vi "AB_860_900_Project_EXE_Info.vi"(7 "action":T1, 8 "error in (no error)":errorcluster, 10 "Exe_info in":T2, 11 "Object In":T3) -> (0 "error out":errorcluster, 2 "Exe info out":T2, 3 "Object Out":T3)   [LabVIEW 2020]
uses:
  <resource>/Framework/Providers/API/ItemRef.ctl
  <vilib>/AppBuilder/RW_Project/AB_RW_Project_PropBag_Action.ctl
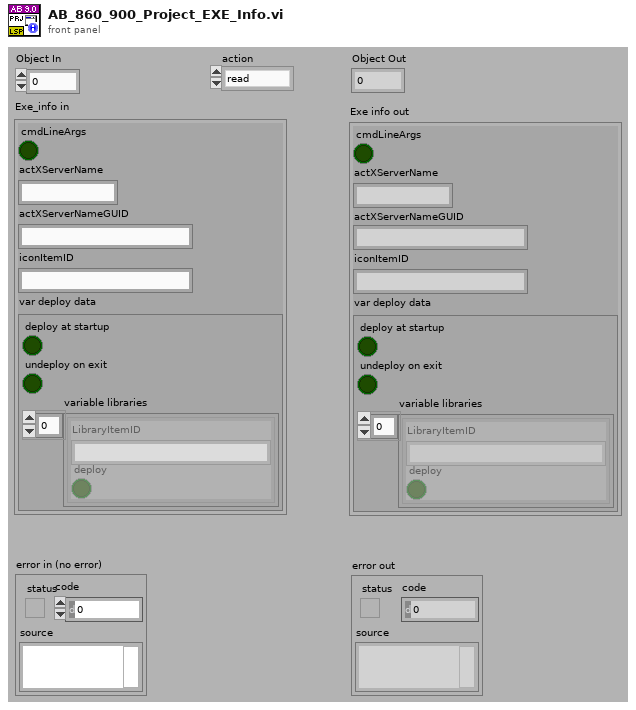
[diagram p1: front panel]
types:
  T1 = typedef "AB_RW_Project_PropBag_Action.ctl" = enum16{"read", "write", "clear", "readPrevious", "writePrevious", "clearPrevious"}
  T2 = cluster{"cmdLineArgs":bool, "actXServerName":string, "actXServerNameGUID":string, "iconItemID":string, "var deploy data":cluster{"deploy at startup":bool, "undeploy on exit":bool, "variable libraries":cluster{"LibraryItemID":string, "deploy":bool}[]}}
  T3 = typedef "ItemRef.ctl" = u64
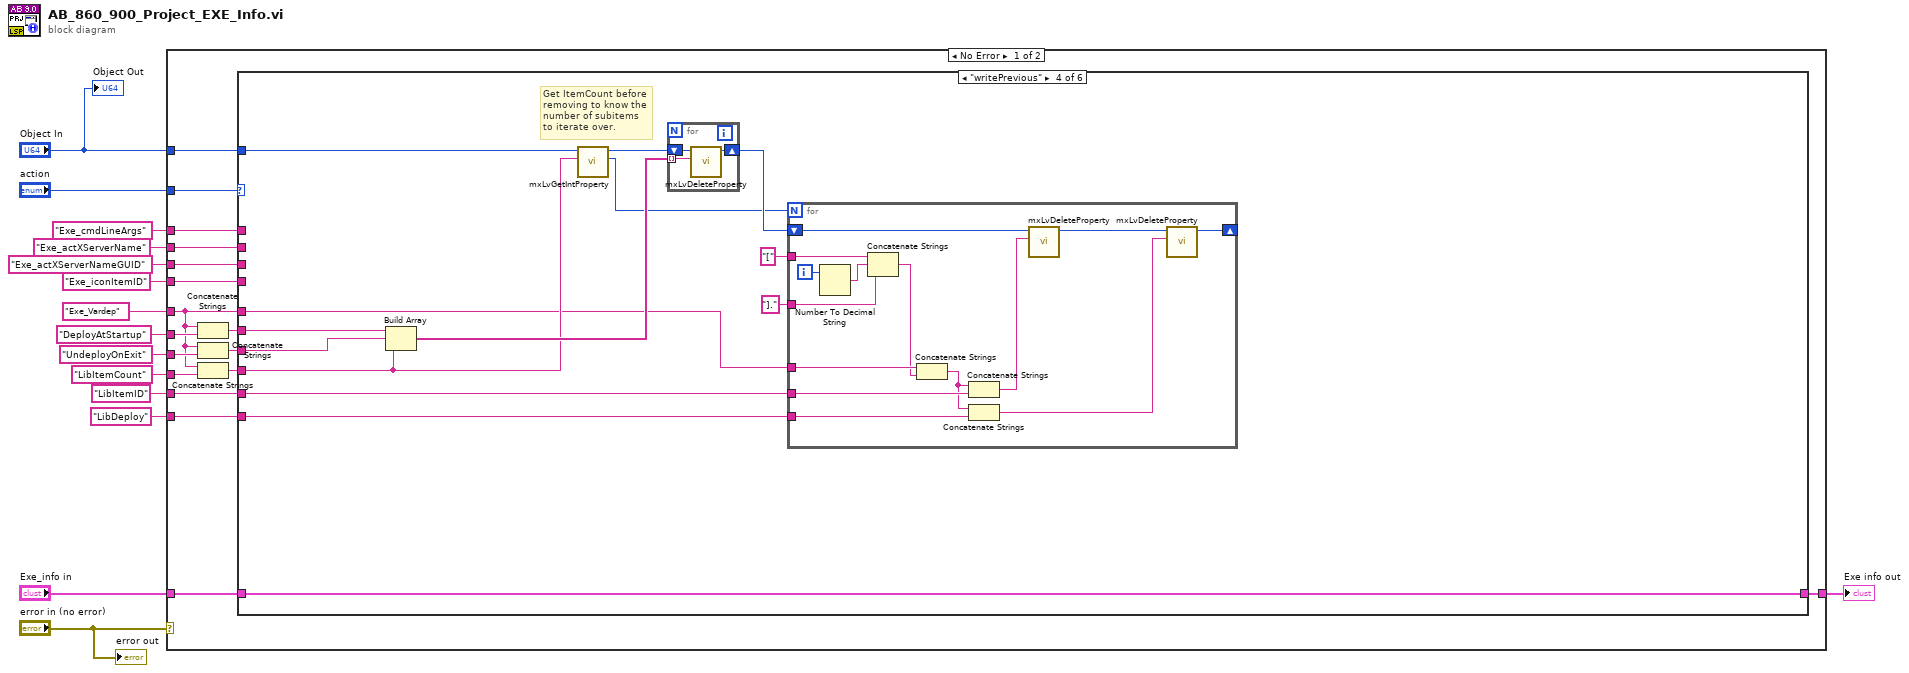
[diagram p0: block diagram]
diagram:
  n1 = case shown="No Error" "error in (no error)" {
    tunnel: "Object In" -> [w30 _]
    tunnel: [w32 _] -> w13
    tunnel: "Exe_cmdLineArgs" -> [w31 _]
    tunnel: "Exe_actXServerName" -> [w29 _]
    tunnel: "Exe_actXServerNameGUID" -> [w28 _]
    tunnel: "Exe_info in" -> [w27 _]
    tunnel: "action" -> [w26 _]
    tunnel: "Exe_iconItemID" -> [w25 _]
    tunnel: "Exe_Vardep" -> [w18 _]
    tunnel: "DeployAtStartup" -> [w21 _]
    tunnel: "UndeployOnExit" -> [w20 _]
    tunnel: "LibItemCount" -> [w19 _]
    tunnel: "LibItemID" -> [w24 _]
    tunnel: "LibDeploy" -> [w23 _]
    frame No Error {
      n2 = Concatenate Strings(w18, w21) -> (w17:string)
      n3 = Concatenate Strings(w18, w20) -> (w22:string)
      n4 = Concatenate Strings(w18, w19) -> (w16:string)
      n5 = case shown="\"writePrevious\"" w26 {
        tunnel: [w33 w34 w35 w49 w67 w68] -> w32
        tunnel: w31 -> [_ _ _ _ _ _]
        tunnel: w30 -> [_ _ _ w36 _ _]
        tunnel: w29 -> [_ _ _ _ _ _]
        tunnel: w28 -> [_ _ _ _ _ _]
        tunnel: w27 -> [w33 w34 w35 w49 w67 w68]
        tunnel: w25 -> [_ _ _ _ _ _]
        tunnel: w18 -> [_ _ _ w39 _ _]
        tunnel: w17 -> [_ _ _ w47 _ _]
        tunnel: w22 -> [_ _ _ w46 _ _]
        tunnel: w16 -> [_ _ _ w44 _ _]
        tunnel: w24 -> [_ _ _ w38 _ _]
        tunnel: w23 -> [_ _ _ w37 _ _]
        frame "read" {
        }
        frame "write" {
        }
        frame "clear" {
        }
        frame "writePrevious" {
          # "Get ItemCount before removing to know the number of subitems to iterate over."
          n6 = Build Array(w47, w46, w44) -> (w45:string[])
          n7 = call <resource>:"mxLvGetIntProperty.vi"("Tag"=w44, "Item"=w36) -> ("Value"=w40:i32, "Item"=w48:T3)  [unwired: 1 in, 7 out]
          n8 = for {
            tunnel: w45 -> [w65] mode=indexing
            shift-right: [w64] -> w41
            shift-left: w48 -> [w66]
            n9 = call <resource>:"mxLvDeleteProperty.vi"("Tag"=w65, "Item"=w66) -> ("Item"=w64:T3)  [unwired: 1 in, 8 out]
          }
          n10 = for {
            N: w40 -> [_]
            shift-right: [w63] -> _
            shift-left: w41 -> [w62]
            tunnel: "[" -> [w59]
            tunnel: "]." -> [w58]
            tunnel: w39 -> [w57]
            tunnel: w38 -> [w55]
            tunnel: w37 -> [w54]
            i -> [w60]
            n11 = Number To Decimal String(number=w60) -> (decimal integer string=w61:string)  [unwired: 1 out]
            n12 = Concatenate Strings(w59, w61, w58) -> (w56:string)
            n13 = Concatenate Strings(w57, w56) -> (w51:string)
            n14 = Concatenate Strings(w51, w55) -> (w53:string)
            n15 = Concatenate Strings(w51, w54) -> (w52:string)
            n16 = call <resource>:"mxLvDeleteProperty.vi"("Tag"=w53, "Item"=w62) -> ("Item"=w50:T3)  [unwired: 1 in, 8 out]
            n17 = call <resource>:"mxLvDeleteProperty.vi"("Tag"=w52, "Item"=w50) -> ("Item"=w63:T3)  [unwired: 1 in, 8 out]
          }
        }
        frame "readPrevious" {
        }
        frame "clearPrevious" {
        }
      }
    }
    frame Error {
    }
  }
  "Exe info out" <- w13
  "Object Out" <- "Object In"
  "error out" <- "error in (no error)"
